vi "actions.vi"(8 "Error In":errorcluster, 11 "QWidget In":refnum<class "QWidget.lvclass">) -> (0 "Error Out":errorcluster, 2 "Value":refnum<class "QAction.lvclass">[](array[class]), 3 "QWidget Out":refnum<class "QWidget.lvclass">)   [LabVIEW 2014, in "QWidget.lvclass"]
doc: "LabVIEW-specific documentation is not yet available. See <b>https://doc.qt.io/qt-5/qwidget.html#actions</b>"
uses:
  QWidget.lvclass
  QAction/QAction.lvclass
  LQ Core/LQIdentity/LQIdentity.lvclass/LQIdentity.ctl
  LQ Core/LQ Core.lvlib
  LQ Core/LQIdentity/LQIdentity.lvclass
  LQ Core/LQCoreEngine/LQCoreEngine.lvclass
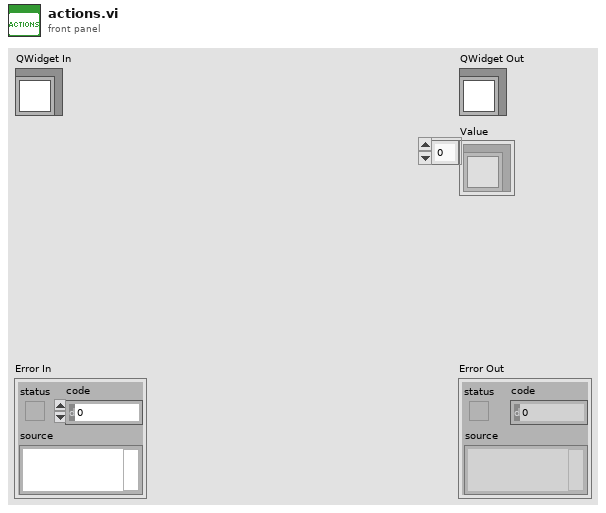
[diagram p1: front panel]
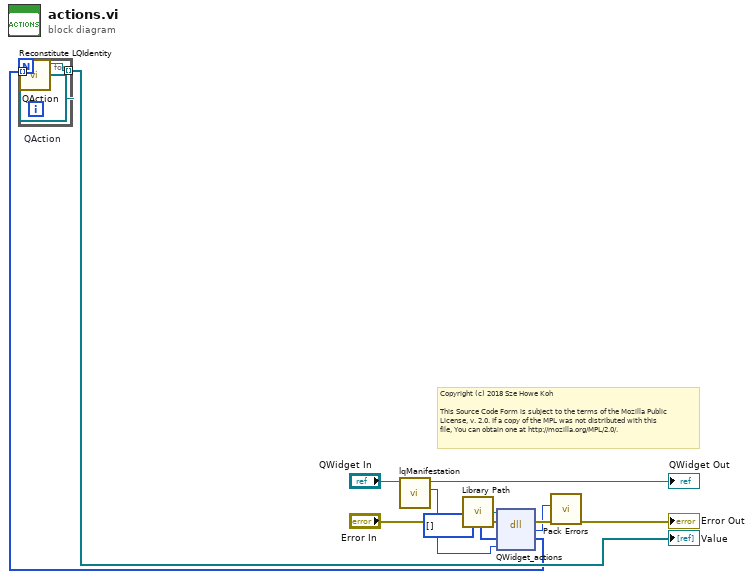
[diagram p0: block diagram]
diagram:
  # "Copyright (c) 2018 Sze Howe Koh\n\nThis Source Code Form is subject to the terms of the Mozilla Public\nLicense, v. 2.0. If a copy of the MPL was not distributed with this\nfile, You can obtain one at http://mozilla.org/MPL/2.0/."
  n1 = call "lqManifestation.vi"("LQIdentity in"="QWidget In") -> ("Manifestation"=w7:u64, "LQIdentity out"=→"QWidget Out":refnum<class "QWidget.lvclass">)  [unwired: 9 in]
  n2 = call "Library Path.vi"() -> ("Library Path"=w8:path)
  n3 = dll-call lib="?" fn="QWidget_actions"(path in=w8, error in="Error In", "_retVal"=u64[] [] ("retVal"), "_instance"=w7) -> (error out=w5:errorcluster, w3:i32, "_retVal"=w1:u64[])  [unwired: 2 in, 1 out]
  n4 = for {
    tunnel: [w14] -> w2 mode=indexing
    tunnel: w1 -> [w12] mode=indexing
    w13 = refnum<class "QAction.lvclass"> refnum  # QAction
    n5 = call "Reconstitute LQIdentity.vi"("Manifestation"=w12, "LQIdentity Prototype"=w13) -> ("Reconstituted LQIdentity"=w14:refnum<class "QAction.lvclass">)  [unwired: 8 in, 1 out]
  }
  "Value" <- w2
  n6 = call "Pack Errors.vi"("Error In"=w5, "Error Code"=w3) -> ("Error Out"=→"Error Out":errorcluster)  [unwired: 9 in]
